vi "Mod_OFDM_Examine_Configure_Waveform_Generation.vi"(11 "error in":errorcluster) -> (8 "Config_Waveform":T1={"Phase Continous \nWaveform"=FALSE, "Store Waveform\nTo a File"=TRUE, "Generate Waveform"=TRUE, "Store Waveform + \nConfiguration To Files"=FALSE}, 15 "error out":errorcluster)   [LabVIEW 2010]
doc: "This is a dialog VI which allows user to select from the following three options:\n\n1) Phase Continuous Waveform: This generates a phase-continuous OFDM modulated signal which may be used with the arbitrary waveform generator\n\n2) Store Waveform To a Datalog File: Click on the \"Store Waveform to File\" control to store the generated waveform in a Datalog file.\n\n3) Store Waveform + Configuration to Files: Click on the \"Store Waveform + Configuration to Files\" control to store the generated waveform in a Datalog file and the configuration in an .ofm file."
panel:
  in  "Store Waveform + \nConfiguration To Files":bool
  in  "Generate Phase \nContinous Waveform":bool
  in  "Store Waveform\nTo a Datalog File":bool
  in  "Cancel Operation":bool
  in  "OK":bool
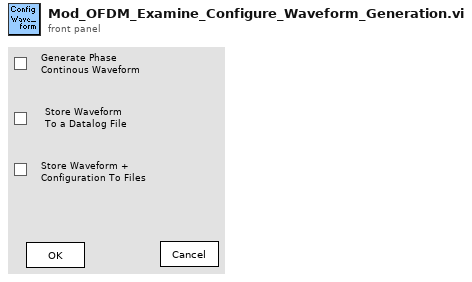
[diagram p1: front panel]
types:
  T1 = cluster{"Phase Continous \nWaveform":bool, "Store Waveform\nTo a File":bool, "Generate Waveform":bool, "Store Waveform + \nConfiguration To Files":bool}
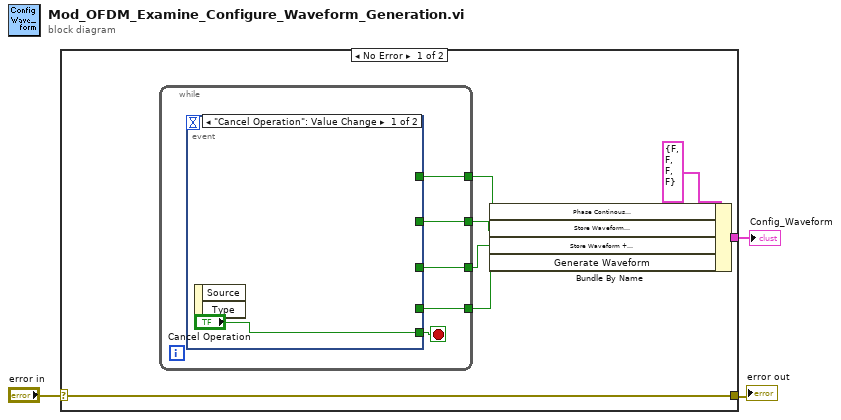
[diagram p0: block diagram]
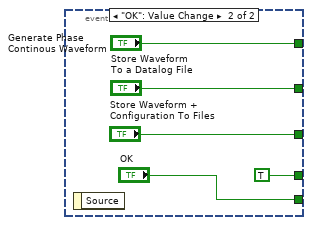
[diagram p2: hidden frame]
diagram:
  n1 = case shown="No Error" "error in" {
    selector: "error in" -> [w10 w22]
    tunnel: [w10 w22] -> w2
    tunnel: [w7 _] -> w1
    frame No Error {
      n2 = while {
        tunnel: [w14] -> w8
        tunnel: [w13] -> w6
        tunnel: [w12] -> w5
        tunnel: [w11] -> w4
        stop <- w15 stop-if-true
        n3 = event shown="[0] \"Cancel Operation\": Value Change" {
          selector: _ -> [_ _]
          dyn-events: _ -> [_ _]
          timeout: _ -> [_ _]
          tunnel: ["Cancel Operation" "OK"] -> w15
          tunnel: [_ "Generate Phase \nContinous Waveform"] -> w13
          tunnel: [_ "Store Waveform\nTo a Datalog File"] -> w12
          tunnel: [_ TRUE ("Store Waveform\nTo a File")] -> w14
          tunnel: [_ "Store Waveform + \nConfiguration To Files"] -> w11
          event "Cancel Operation": Value Change {
            n4 = event-data() -> ()  [unwired: 1 in, 2 out]
          }
          event "OK": Value Change {
            n5 = event-data() -> ()  [unwired: 1 in, 1 out]
          }
        }
      }
      n6 = Bundle By Name(cluster=T1 {"Phase Continous \nWaveform"=FALSE, "Store Waveform\nTo a File"=FALSE, "Generate Waveform"=FALSE, "Store Waveform + \nConfiguration To Files"=FALSE} ("Config_Waveform"), "Phase Continous \nWaveform"=w6, "Store Waveform\nTo a File"=w5, "Store Waveform + \nConfiguration To Files"=w4, "Generate Waveform"=w8) -> (w7:T1)
    }
    frame Error {
    }
  }
  "error out" <- w2
  "Config_Waveform" <- w1
